vi "SingleMoleculePatternFinder.vi"(0 "Image In":T6, 1 "Settings (GeometricMatching)":T4={"Curve Parameters"={"Extraction Mode"=0, "Edge Threshold"=75, "Edge Filter Size"=1, "Min Length"=25, "Row Search Step Size"=15, "Col Search Step Size"=15, "Max Endpoint Gap"=10, "Closed"=FALSE, "Subpixel"=FALSE}, "Match Mode"={"Rotation"=TRUE, "Scale"=FALSE, "Occlusion"=TRUE, "Reserved"=FALSE, "Reserved"=FALSE, "Reserved"=FALSE}, "Range Settings"=[{"Match Constraints"=0, "Min"=0.0, "Max"=360.0}, {"Match Constraints"=2, "Min"=0.0, "Max"=25.0}], "Number of Matches"=5, "Minimum Match Score"=600.0, "SubPixel Accuracy"=FALSE, "Adv. Geometric Match Options 2"=[{"Setup Data Item"=21, "Item Value"=0.0}, {"Setup Data Item"=22, "Item Value"=1.0}]} {"Curve Parameters"."Extraction Mode" items=["Normal", "Uniform Regions"]; "Curve Parameters"."Edge Filter Size" items=["Fine", "Normal", "Contour Tracing"]; "Curve Parameters"."Max Endpoint Gap" min=0; "Curve Parameters"."Col Search Step Size" min=1 max=255 step=1; "Curve Parameters"."Row Search Step Size" min=1 max=255 step=1; "Curve Parameters"."Min Length" min=0; "Curve Parameters"."Edge Threshold" min=1 max=350 step=1; "Range Settings"."Max" format="%.2f"; "Range Settings"."Min" format="%.2f"; "Range Settings"."Match Constraints" items=["Rotation Angle (degrees)", "Scale Factor (%)", "Occlusion (%)"]; "Adv. Geometric Match Options 2"."Setup Data Item" items=["Curve Extraction Mode", "Curve Edge Threshold", "Curve Edge Filter Size", "Min Curve Length", "Curve Row Search Step Size", "Curve Col Search Step Size", "Curve Max Endpoint Gap", "Extract Closed Curves", "Enable Subpixel Curve Extraction", "Enable Correlation Score", "Enable Subpixel Accuracy", "Subpixel Iterations", "Subpixel Tolerance", "Initial Match List Length", "Enable Target Template Curve Score", "Min Match Separation Distance", "Min Match Separation Angle", "Min Match Separation Scale", "Max Match Overlap", "Enable Coarse Result", "Enable Calibration Support", "Enable Contrast Reversal", "Search Strategy", "Refinement Match Factor", "Subpixel Match Factor"]}, 7 "error in":errorcluster, 9 "Template File Path (GeometricMatching)":path=path "C:/Users/dhaehnel/Desktop/SingleMoleculePatternFinder/Patterns/azimuthal.png") -> (21 "Matches (GeometricMatching)":T5[](array[typedef]) {"Correlation Score" format="%.2f"; "Target Template Curve Score" format="%.2f"; "Template Target Curve Score" format="%.2f"; "Bounding Box"."y" format="%.2f"; "Bounding Box"."x" format="%.2f"; "Position"."y" format="%.2f"; "Position"."x" format="%.2f"; "Score" format="%.2f"; "Scale" format="%.2f"; "Angle" format="%.2f"; "Occlusion %" format="%.2f"}, 23 "Number of Matches (GeometricMatching)":i32, 27 "error out":errorcluster)   [LabVIEW 2013]
uses:
  <vilib>/vision/Image Controls.llb/IMAQ Image.ctl
  <vilib>/vision/Pattern Matching.llb/IMAQ GM Match Report.ctl
  <vilib>/vision/Pattern Matching.llb/IMAQ Curve Parameters.ctl
  <vilib>/vision/Pattern Matching.llb/IMAQ Match Range Setting.ctl
  <vilib>/vision/NI_Vision_Development_Module.lvlib
panel:
  in  "ROI Descriptor (GeometricMatching)":T1={"Global Rectangle"=[20, 20, 1045, 788], "Contours"=[{"ID"=enum."External", "Type"=3, "Coordinates"=[20, 20, 1045, 788]}]} {"Contours"."Type" items=["No Selection", "Point", "Line", "Rectangle", "Oval", "Polygon", "Freehand Region", "Annulus", "Unused2", "Unused3", "Broken Line", "Freehand Line", "Rotated Rectangle"]}
  out "Calibrated Matches (GeometricMatching)":T5[](array[typedef]) {"Correlation Score" format="%.2f"; "Target Template Curve Score" format="%.2f"; "Template Target Curve Score" format="%.2f"; "Bounding Box"."y" format="%.2f"; "Bounding Box"."x" format="%.2f"; "Position"."y" format="%.2f"; "Position"."x" format="%.2f"; "Score" format="%.2f"; "Scale" format="%.2f"; "Angle" format="%.2f"; "Occlusion %" format="%.2f"}
  out "Image Out":T6
  # "Range"
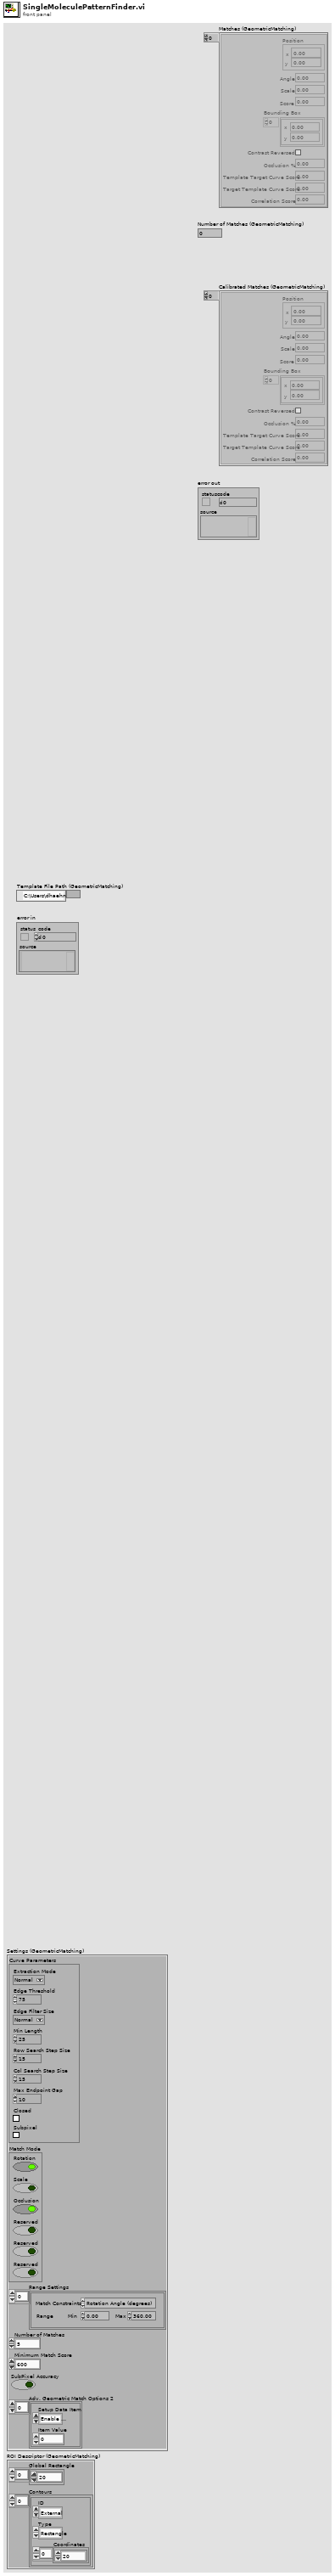
[diagram p1: front panel]
types:
  T1 = cluster{"Global Rectangle":i32[], "Contours":cluster{"ID":enum32{"External", "Internal"}, "Type":u32, "Coordinates":i32[]}[]}
  T2 = typedef "IMAQ Curve Parameters.ctl" = cluster{"Extraction Mode":u32, "Edge Threshold":i32, "Edge Filter Size":u32, "Min Length":i32, "Row Search Step Size":i32, "Col Search Step Size":i32, "Max Endpoint Gap":i32, "Closed":bool, "Subpixel":bool}
  T3 = typedef "IMAQ Match Range Setting.ctl" = cluster{"Match Constraints":u32, "Min":dbl, "Max":dbl}
  T4 = cluster{"Curve Parameters":T2, "Match Mode":cluster{"Rotation":bool, "Scale":bool, "Occlusion":bool, "Reserved":bool, "Reserved":bool, "Reserved":bool}, "Range Settings":T3[], "Number of Matches":i32, "Minimum Match Score":sgl, "SubPixel Accuracy":bool, "Adv. Geometric Match Options 2":cluster{"Setup Data Item":u16, "Item Value":dbl}[]}
  T5 = typedef "IMAQ GM Match Report.ctl" = cluster{"Position":cluster{"x":sgl, "y":sgl}, "Angle":sgl, "Scale":sgl, "Score":sgl, "Bounding Box":cluster{"x":sgl, "y":sgl}[], "Contrast Reversed":bool, "Occlusion %":sgl, "Template Target Curve Score":sgl, "Target Template Curve Score":sgl, "Correlation Score":sgl}
  T6 = typedef "IMAQ Image.ctl" = refnum<image>
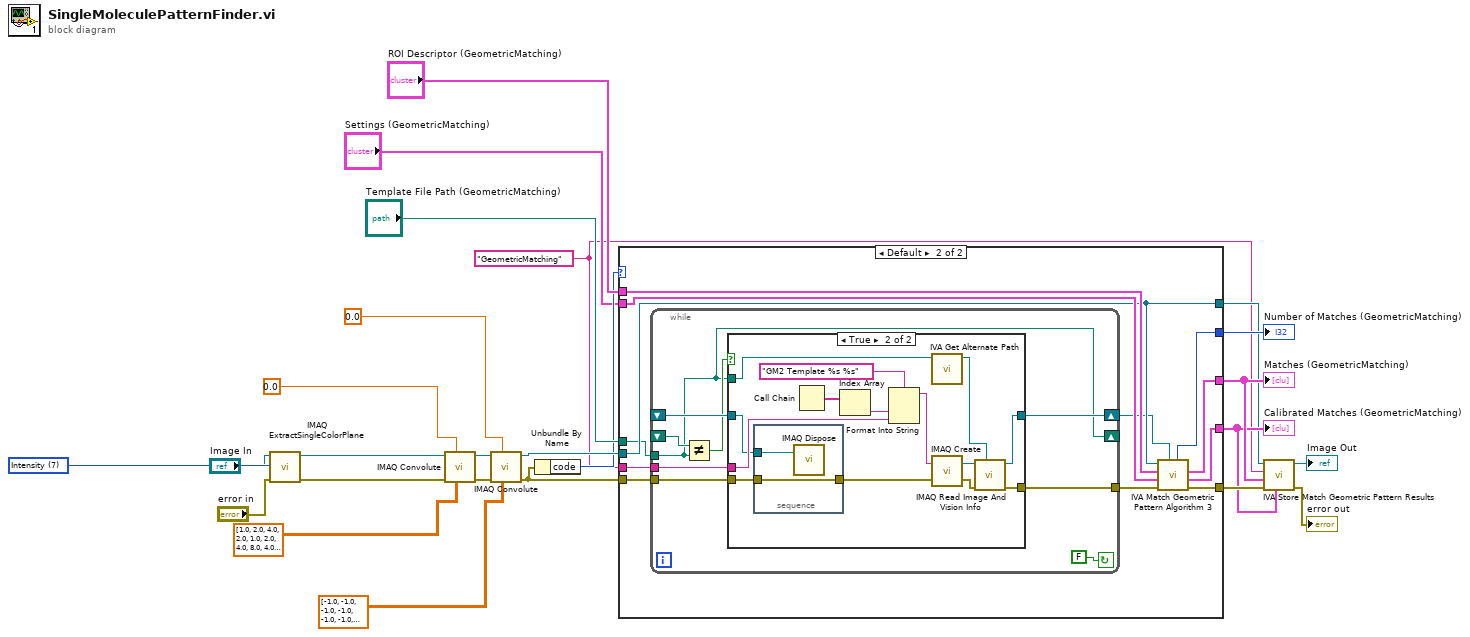
[diagram p0: block diagram]
diagram:
  w25 = 7 items=["Red", "Green", "Blue", "Hue", "Saturation", "Luminance", "Value", "Intensity"] ("Color Plane (IntensityExtraction)")
  w1 = "GeometricMatching" ("Step Name")
  n1 = call "IMAQ ExtractSingleColorPlane"("Color Plane"=w25, "error in (no error)"="error in", "Image Src"="Image In") -> ("error out"=w20:errorcluster, "Image Dst Out"=w21:T6)  [unwired: 1 in, 6 out]
  n2 = call "IMAQ Convolute"("Kernel"=sgl[][] [[1.0, 2.0, 4.0, 2.0, 1.0], [2.0, 4.0, 8.0, 4.0, 2.0], [4.0, 8.0, 16.0, 8.0, 4.0], [2.0, 4.0, 8.0, 4.0, 2.0], [1.0, 2.0, 4.0, 2.0, 1.0]] ("Kernel (SmothingGaussian)"), "Divider (kernel sum)"=sgl 0.0 ("Divider (SmothingGaussian)"), "error in (no error)"=w20, "Image Src"=w21) -> ("error out"=w16:errorcluster, "Image Dst Out"=w17:T6)  [unwired: 3 in, 3 out]
  n3 = call "IMAQ Convolute"("Kernel"=sgl[][] [[-1.0, -1.0, -1.0, -1.0, -1.0], [-1.0, -1.0, -1.0, -1.0, -1.0], [-1.0, -1.0, 30.0, -1.0, -1.0], [-1.0, -1.0, -1.0, -1.0, -1.0], [-1.0, -1.0, -1.0, -1.0, -1.0]] ("Kernel (Convolution)"), "Divider (kernel sum)"=sgl 0.0 ("Divider (Convolution)"), "error in (no error)"=w16, "Image Src"=w17) -> ("error out"=w5:errorcluster, "Image Dst Out"=w12:T6)  [unwired: 3 in, 3 out]
  n4 = Unbundle By Name(w5) -> ("code"=w4:i32)
  n5 = case shown="Default" w4 {
    tunnel: "Template File Path (GeometricMatching)" -> [_ w28]
    tunnel: w5 -> [_ w29]
    tunnel: "Settings (GeometricMatching)" -> [_ w38]
    tunnel: "ROI Descriptor (GeometricMatching)" -> [_ w37]
    tunnel: w12 -> [w26 w32]
    tunnel: [_ w36] -> w10
    tunnel: [_ w35] -> w8
    tunnel: [_ w34] -> w7
    tunnel: [_ w33] -> w6
    tunnel: [w26 w32] -> w3
    tunnel: w1 -> [_ w27]
    frame -1074396199, -1074396198 {
      # "Discard Coordinate System Error"
    }
    frame Default {
      n6 = while {
        shift-right: [w47] -> w30
        shift-left: _ -> [w46]
        tunnel: [w44] -> w31
        tunnel: w29 -> [w43]
        tunnel: w28 -> [w39]
        tunnel: w27 -> [w42]
        shift-right: [w39] -> _
        shift-left: _ -> [w41]
        stop <- FALSE continue-if-true
        n7 = Not Equal?(x=w41, y=w39) -> (x != y?=w40:bool)
        n8 = case shown="True" w40 {
          tunnel: [w49 w61] -> w47
          tunnel: w46 -> [w49 w53]
          tunnel: [w48 w58] -> w44
          tunnel: w43 -> [w48 w54]
          tunnel: w42 -> [_ w55]
          tunnel: w39 -> [_ w51]
          frame False {
          }
          frame True {
            n9 = stacked-sequence {
              tunnel: w54 -> [w65]
              tunnel: w53 -> [w64]
              tunnel: [w65] -> w52
              frame #0 {
                n10 = call "IMAQ Dispose"("Image"=w64) -> ()  [unwired: 2 in, 4 out]
              }
            }
            n11 = Call Chain() -> (call chain=w57:string[])
            n12 = Index Array(array=w57) -> (element=w56:string)  [unwired: 1 in]
            n13 = Format Into String(format string="GM2 Template %s %s" ("Image Name"), w56, w55) -> (resulting string=w63:string)  [unwired: 2 in, 1 out]
            n14 = call <vilib>:"IVA Get Alternate Path.vi"("Path In"=w51) -> ("Path Out"=w50:path)  [unwired: 10 out]
            n15 = call "IMAQ Create"("Image Name"=w63, "error in (no error)"=w52) -> ("New Image"=w60:T6, "error out"=w59:errorcluster)  [unwired: 2 in, 1 out]
            n16 = call "IMAQ Read Image And Vision Info"("File Path"=w50, "error in (no error)"=w59, "Image"=w60) -> ("error out"=w58:errorcluster, "Image Out"=w61:T6)  [unwired: 1 in, 6 out]
          }
        }
      }
      n17 = call <vilib>:"IVA Match Geometric Pattern Algorithm 3.vi"("Template"=w30, "error in (no error)"=w31, "Settings"=w38, "ROI Descriptor"=w37, "Image"=w32) -> ("error out"=w36:errorcluster, "Calibrated Matches"=w34:T5[], "Matches"=w35:T5[], "Number of Matches"=w33:i32)  [unwired: 3 out]
    }
  }
  "Matches (GeometricMatching)" <- w8
  "Number of Matches (GeometricMatching)" <- w6
  "Calibrated Matches (GeometricMatching)" <- w7
  n18 = call <vilib>:"IVA Store Match Geometric Pattern Results.vi"("Calibrated Matches"=w7, "error in (no error)"=w10, "Matches"=w8, "Step Name"=w1, "Image in"=w3) -> ("error out"=→"error out":errorcluster, "Image dup"=→"Image Out":T6)  [unwired: 5 out]
